vi "princess_mode.vi"(8 "error out":errorcluster, 9 "plots":refnum<vi>, 10 "experiments":refnum<vi>, 11 "VI in":refnum<vi>) -> (0 "error out 2":errorcluster)   [LabVIEW 2018]
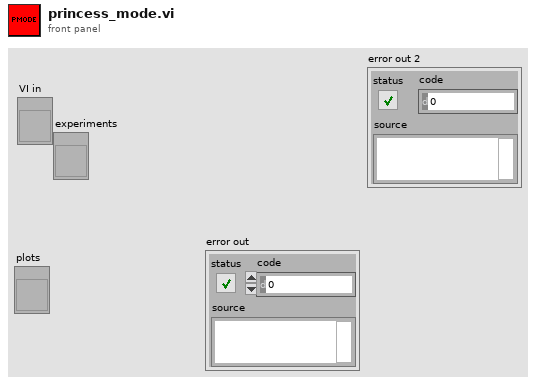
[diagram p1: front panel]
types:
  T1 = typedef "imagedata.ctl" = cluster{"image type":i32, "image depth":i32, "image":u8[], "mask":u8[], "colors":u32[], "Rectangle":cluster{"left":i16, "top":i16, "right":i16, "bottom":i16}}
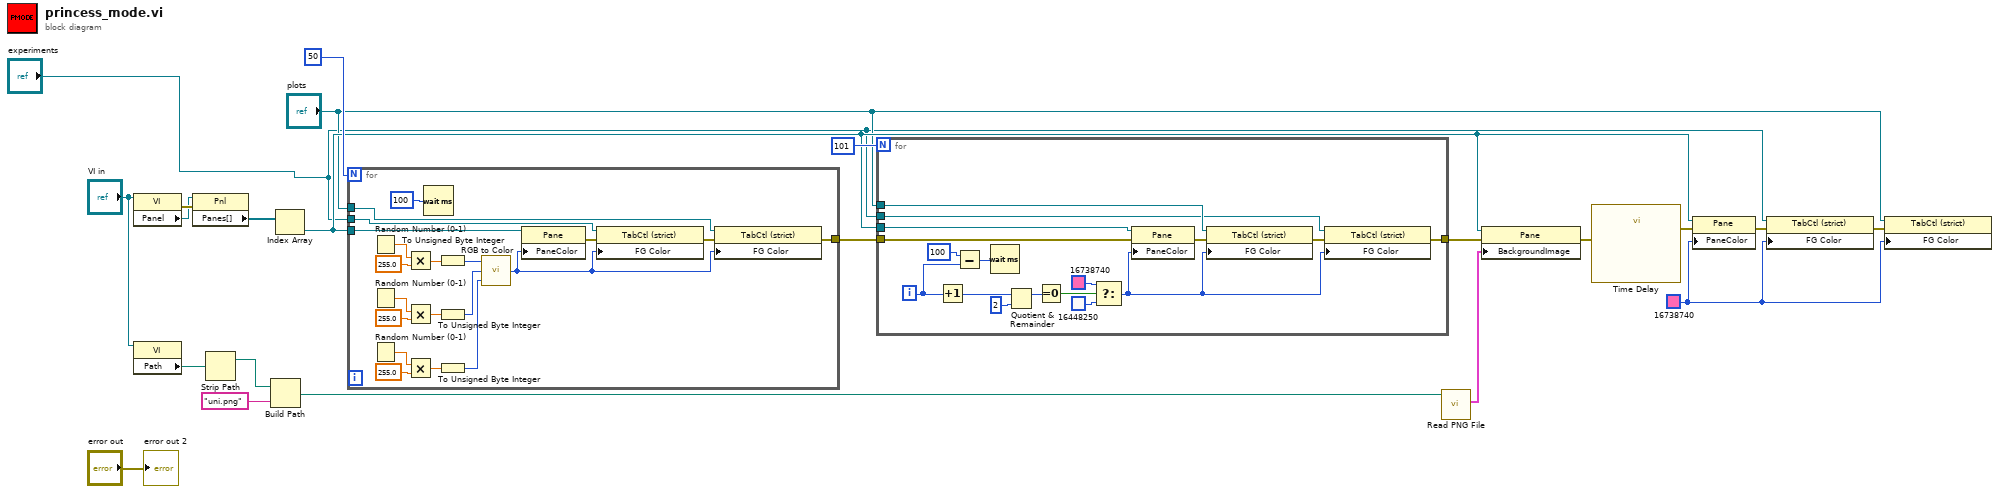
[diagram p0: block diagram]
diagram:
  w2 = u32 16738740
  n1 = property class="VI"(reference="VI in") -> (error out=w18:errorcluster, "Panel"=w7:refnum<vi>)  [unwired: 1 in, 1 out]
  n2 = property class="VI"(reference="VI in") -> ("Path"=w16:path)  [unwired: 1 in, 2 out]
  n3 = property class="Pnl"(reference=w7, error in=w18) -> ("Panes[]"=w10:refnum<vi>[])  [unwired: 2 out]
  n4 = Strip Path(path=w16) -> (stripped path=w15:path)  [unwired: 1 out]
  n5 = Build Path(base path=w15, name or relative path="uni.png") -> (appended path=w13:path)
  n6 = Index Array(array=w10) -> (element=w9:refnum<vi>)  [unwired: 1 in]
  n7 = for {
    N: 50 -> [_]
    tunnel: [w26] -> w21
    tunnel: w9 -> [w29]
    tunnel: "experiments" -> [w25]
    tunnel: "plots" -> [w24]
    n8 = Random Number (0-1)() -> (number: 0 to 1=w42:dbl)
    n9 = Random Number (0-1)() -> (number: 0 to 1=w39:dbl)
    n10 = Random Number (0-1)() -> (number: 0 to 1=w36:dbl)
    n11 = Multiply(x=w42, y=255.0) -> (x*y=w40:dbl)
    n12 = Multiply(x=w39, y=255.0) -> (x*y=w37:dbl)
    n13 = Multiply(x=w36, y=255.0) -> (x*y=w34:dbl)
    n14 = Wait (ms)(milliseconds to wait=u32 100) -> ()  [unwired: 1 out]
    n15 = To Unsigned Byte Integer(number=w40) -> (unsigned 8bit integer=w33:u8)
    n16 = To Unsigned Byte Integer(number=w37) -> (unsigned 8bit integer=w32:u8)
    n17 = To Unsigned Byte Integer(number=w34) -> (unsigned 8bit integer=w31:u8)
    n18 = call <vilib>:"RGB to Color.vi"("B"=w31, "G"=w32, "R"=w33) -> ("Color"=w23:u32)
    n19 = property class="Pane"(reference=w29, "PaneColor"=w23) -> (error out=w28:errorcluster)  [unwired: 1 in, 1 out]
    n20 = property class="TabCtl (strict)"(reference=w25, error in=w28, "FG Color"=w23) -> (error out=w27:errorcluster)  [unwired: 1 out]
    n21 = property class="TabCtl (strict)"(reference=w24, error in=w27, "FG Color"=w23) -> (error out=w26:errorcluster)  [unwired: 1 out]
  }
  n22 = for {
    N: 101 -> [_]
    tunnel: w21 -> [w50]
    tunnel: w9 -> [w49]
    tunnel: [w46] -> w6
    tunnel: "plots" -> [w44]
    tunnel: "experiments" -> [w43]
    i -> [w53]
    n23 = Increment(x=w53) -> (x+1=w58:i32)
    n24 = Subtract(x=u32 100 ("milliseconds to wait"), y=w53) -> (x-y=w52:u32)
    n25 = Wait (ms)(milliseconds to wait=w52) -> ()  [unwired: 1 out]
    n26 = Quotient & Remainder(x=w58, y=2) -> (x-y*floor(x/y)=w56:i32)  [unwired: 1 out]
    n27 = Equal To 0?(x=w56) -> (x = 0?=w55:bool)
    n28 = Select(t=u32 16738740, s=w55, f=u32 16448250) -> (s? t:f=w45:u32)
    n29 = property class="Pane"(reference=w49, error in=w50, "PaneColor"=w45) -> (error out=w47:errorcluster)  [unwired: 1 out]
    n30 = property class="TabCtl (strict)"(reference=w44, error in=w47, "FG Color"=w45) -> (error out=w48:errorcluster)  [unwired: 1 out]
    n31 = property class="TabCtl (strict)"(reference=w43, error in=w48, "FG Color"=w45) -> (error out=w46:errorcluster)  [unwired: 1 out]
  }
  n32 = call <vilib>:"Read PNG File.vi"("path to PNG file"=w13) -> ("image data"=w22:T1)  [unwired: 8 in, 2 out]
  n33 = property on="Property Node" class="Pane"(reference=w9, error in=w6, "BackgroundImage"=w22) -> (error out=w12:errorcluster)  [unwired: 1 out]
  n34 = call "Time Delay"("error in (no error)"=w12) -> ("error out"=w11:errorcluster)  [unwired: 10 in]
  n35 = property class="Pane"(reference=w9, error in=w11, "PaneColor"=w2) -> (error out=w4:errorcluster)  [unwired: 1 out]
  n36 = property class="TabCtl (strict)"(reference="experiments", error in=w4, "FG Color"=w2) -> (error out=w5:errorcluster)  [unwired: 1 out]
  n37 = property class="TabCtl (strict)"(reference="plots", error in=w5, "FG Color"=w2) -> ()  [unwired: 2 out]
  "error out 2" <- "error out"
